vi "Find EHL Event Structure.vi"(8 "error in (no error)":errorcluster, 11 "VI Ref in":refnum<vi>) -> (0 "error out":errorcluster, 1 "Found?":bool, 2 "EHL Event Structure":refnum<vi>, 3 "VI Ref out":refnum<vi>)   [LabVIEW 2017, in "Open DQMH Request Message Diagram.lvlib"]
doc: "Retruns the DQMH Event Structure reference of the DQMH Module Main VI."
uses:
  <vilib>/Utility/traverseref.llb/TRef TravTarget.ctl
  Open DQMH Request Message Diagram.lvlib
  <vilib>/Utility/traverseref.llb/VI Scripting - Traverse.lvlib
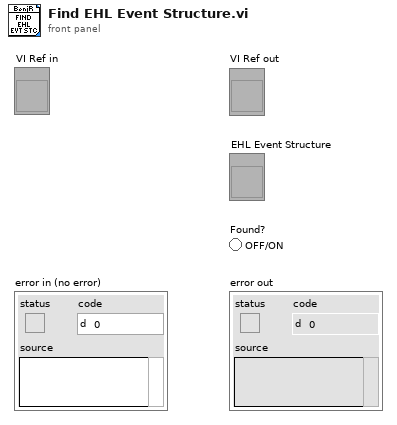
[diagram p1: front panel]
types:
  T1 = typedef "TRef TravTarget.ctl" = enum16{"FP", "BD", "Other"}
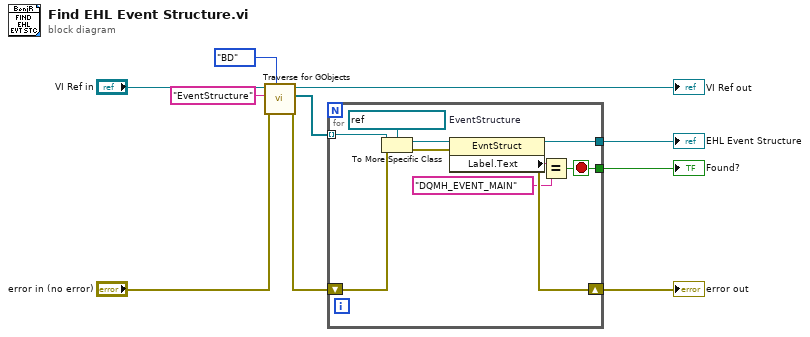
[diagram p0: block diagram]
diagram:
  n1 = call <vilib>:"Traverse for GObjects.vi"("Traverse Target"=TRef_TravTarget."BD", "error in (no error)"="error in (no error)", "Class Name"="EventStructure", "VI Refnum"="VI Ref in") -> ("error out"=w8:errorcluster, "References"=w4:refnum<vi>[], "dup VI Refnum"=→"VI Ref out":refnum<vi>)  [unwired: 4 in, 1 out]
  n2 = for {
    tunnel: w4 -> [w20] mode=indexing
    tunnel: [w15] -> w5
    shift-right: [w14] -> w7
    shift-left: w8 -> [w13]
    tunnel: [w12] -> w10
    stop <- w12 stop-if-true
    w18 = refnum<vi> refnum  # EventStructure
    n3 = To More Specific Class(target class=w18, reference=w20, error in=w13) -> (specific class reference=w19:refnum<vi>, error out=w17:errorcluster)
    n4 = property class="EvntStruct"(reference=w19, error in=w17) -> (reference out=w15:refnum<vi>, error out=w14:errorcluster, "Label.Text"=w16:string)
    n5 = Equal?(x=w16, y="DQMH_EVENT_MAIN" ("Class Name")) -> (x = y?=w12:bool)
  }
  "Found?" <- w10
  "error out" <- w7
  "EHL Event Structure" <- w5
